vi "test.vi"() -> ()   [LabVIEW 2011]
panel:
  out "x << y":i16
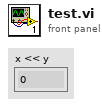
[diagram p1: front panel]
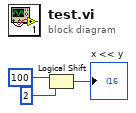
[diagram p0: block diagram]
diagram:
  n1 = Logical Shift(y=i16 100, x=i16 2) -> (x << y=→"x << y":i16)
